vi "global API.vi"() -> ()   [LabVIEW 2020]
panel:
  in  "Port":i32=5555
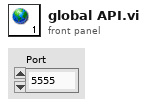
[diagram p1: front panel]
diagram:
